vi "RSZVB Read Instrument Data.vi"(8 "error in (no error)":errorcluster {"code" format="%.0x"}, 10 "Number Bytes To Read (50)":i32=50, 11 "VISA session":refnum<visa-resource-name>) -> (0 "error out":errorcluster {"code" format="%.0x"}, 1 "NumBytes Read":i32, 2 "Read Buffer":string, 3 "dup VISA session":refnum<visa-resource-name>)   [LabVIEW 2011]
doc: "This VI reads data from the instrument's output buffer and returns it to the specified variable in memory.\n\nNotes:\n\n(1) Because the instrument may return both numeric and text data in response to queries this VI returns the data in string format.\n\n(2) If valid data is not available at the instrument's output buffer when this VI is called the instrument will hang up and the function will not return until it times out. If the time-out is disabled this function will hang indefinitely and it may be necessary to reboot the computer to break out."
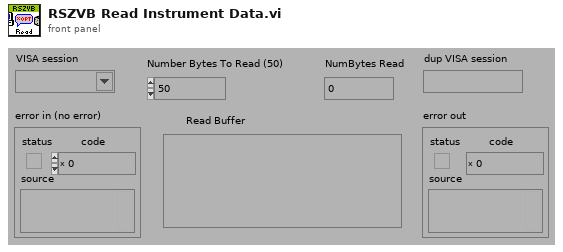
[diagram p1: front panel]
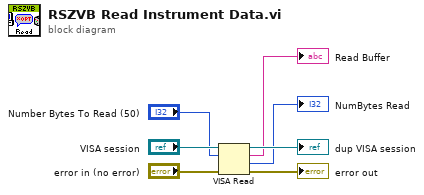
[diagram p0: block diagram]
diagram:
  n1 = VISA Read(VISA resource name="VISA session", byte count="Number Bytes To Read (50)", error in (no error)="error in (no error)") -> (VISA resource name out=→"dup VISA session":refnum<visa-resource-name>, read buffer=→"Read Buffer":string, return count=→"NumBytes Read":u32, error out=→"error out":errorcluster)
